vi "LVDimInterface.test ping pong client.vi"() -> ()   [LabVIEW 2015, in "LVDimInterface.lvlib"]
doc: "This is an example of a DIM client receiving service data via a message queue."
uses:
  LVDimInterface.lvlib
  LVDimInterface.dim service type.ctl
  LVDimInterface.dic_info_service_queue.vi
panel:
  out "error out":errorcluster
  in  "commandName":string="testCommand"
  out "callBackID":i32
  out "no link":bool
  out "serviceData":i32
  out "serviceSize":i32
  in  "serviceName":string="testBuffer"
  out "receivedCounter":i32
  in  "stop":bool
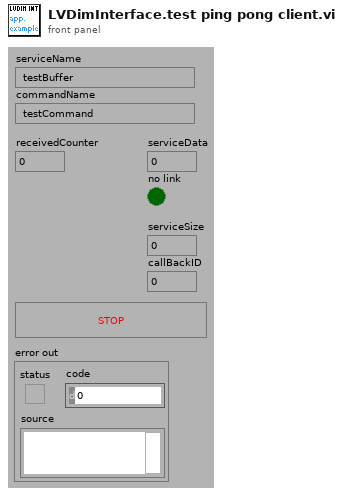
[diagram p1: front panel]
types:
  T1 = typedef "LVDimInterface.lvlib/LVDimInterface.dim service type.ctl" = u16
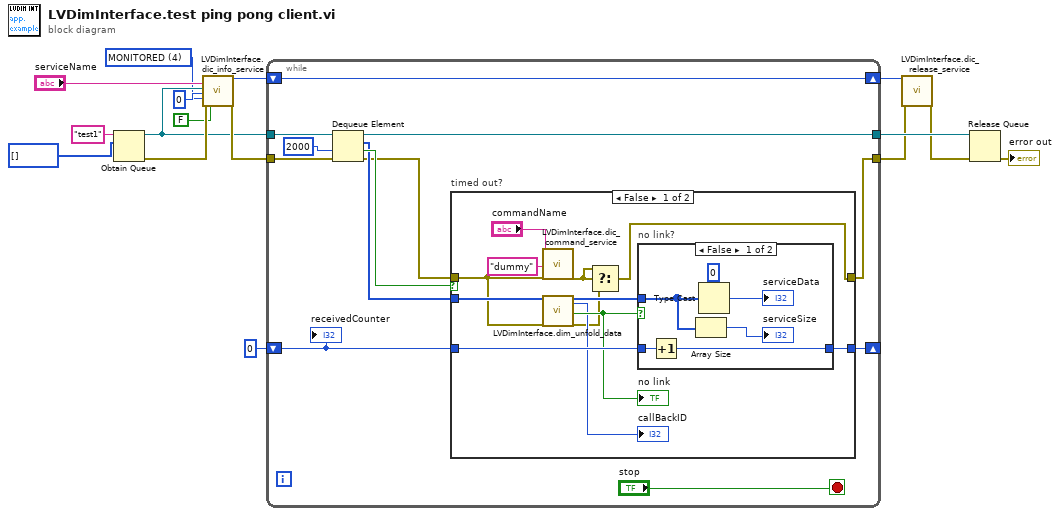
[diagram p0: block diagram]
diagram:
  w3 = T1 4 items=["ONCE_ONLY"=1, "TIMED"=2, "MONITORED"=4] ("serviceType")
  n1 = Obtain Queue(name (unnamed)="test1", element data type=i8[] []) -> (queue out=w5:refnum<queue>, error out=w12:errorcluster)  [unwired: 3 in, 1 out]
  n2 = call-poly "LVDimInterface.dic_info_service.vi"("serviceName"="serviceName", "queueRef"=w5, "timeout [s]"=0, "serviceType"=w3, "error in (no error)"=w12, "stamped"=FALSE) -> ("callBackID"=w15:i32, "error out"=w11:errorcluster)  [unwired: 12 in]
  n3 = while {
    tunnel: w5 -> [w28]
    tunnel: [w26] -> w14
    shift-right: [w22] -> _
    shift-left: 0 -> [w23]
    tunnel: w11 -> [w21]
    tunnel: [w17] -> w9
    shift-right: [w19] -> w10
    shift-left: w15 -> [w19]
    stop <- "stop" stop-if-true
    n4 = Dequeue Element(queue=w28, timeout in ms (-1)=2000, error in (no error)=w21) -> (queue out=w26:refnum<queue>, element=w20:i8[], timed out?=w25:bool, error out=w18:errorcluster)
    n5 = case "timed out?" shown="False" w25 {
      tunnel: [w39 w49] -> w22
      tunnel: w23 -> [w40 w49]
      tunnel: w20 -> [w37 _]
      tunnel: w18 -> [w32 w48]
      tunnel: [w29 w48] -> w17
      frame False {
        n6 = call "LVDimInterface.dic_command_service.vi"("commandName"="commandName", "data"="dummy", "error in (no error)"=w32) -> ("error out"=w30:errorcluster)  [unwired: 15 in, 1 out]
        n7 = call "LVDimInterface.dim_unfold_data.vi"("rawData"=w37, "error in (no error)"=w32) -> ("data"=w38:i8[], "callBackID"=→"callBackID":i32, "no link"=w36:bool, "error out"=w31:errorcluster)  [unwired: 14 in]
        "no link" <- w36
        n8 = Select(t=w30, s=w30, f=w31) -> (s? t:f=w29:errorcluster)
        n9 = case "no link?" shown="False" w36 {
          tunnel: w40 -> [w46 w47]
          tunnel: [w45 w47] -> w39
          tunnel: w38 -> [w42 _]
          frame False {
            n10 = Increment(x=w46) -> (x+1=w45:i32)
            n11 = Array Size(array=w42) -> (size(s)=→"serviceSize":i32)
            n12 = Type Cast(type=0, x=w42) -> (*(type *) &x=→"serviceData":i32)
          }
          frame True {
          }
        }
      }
      frame True {
      }
    }
    "receivedCounter" <- w23
  }
  n13 = call "LVDimInterface.dic_release_service.vi"("callBackID"=w10, "error in (no error)"=w9) -> ("error out"=w8:errorcluster)  [unwired: 17 in]
  n14 = Release Queue(queue=w14, error in (no error)=w8) -> (error out=→"error out":errorcluster)  [unwired: 1 in, 2 out]
